vi "PictureMaquree.vi"() -> ()   [LabVIEW 2021]
uses:
  Control 1.ctl
  <vilib>/vision/NI_Vision_Development_Module.lvlib
panel:
  out "selected path":path
  in  "Delay Times":u64(knob) scale=1.0..500.0
  out "Original":T1(plugin-control)
  in  "Threshold":i64(slide)=125 scale=0.0..255.0
  out "Output Array":bool[][](array[boolean])
  out "ROI":T1(plugin-control)
  in  "Add Button":bool
  in  "Stop Button":bool
  in  "Pause Button":bool
  in  "Play Button":bool
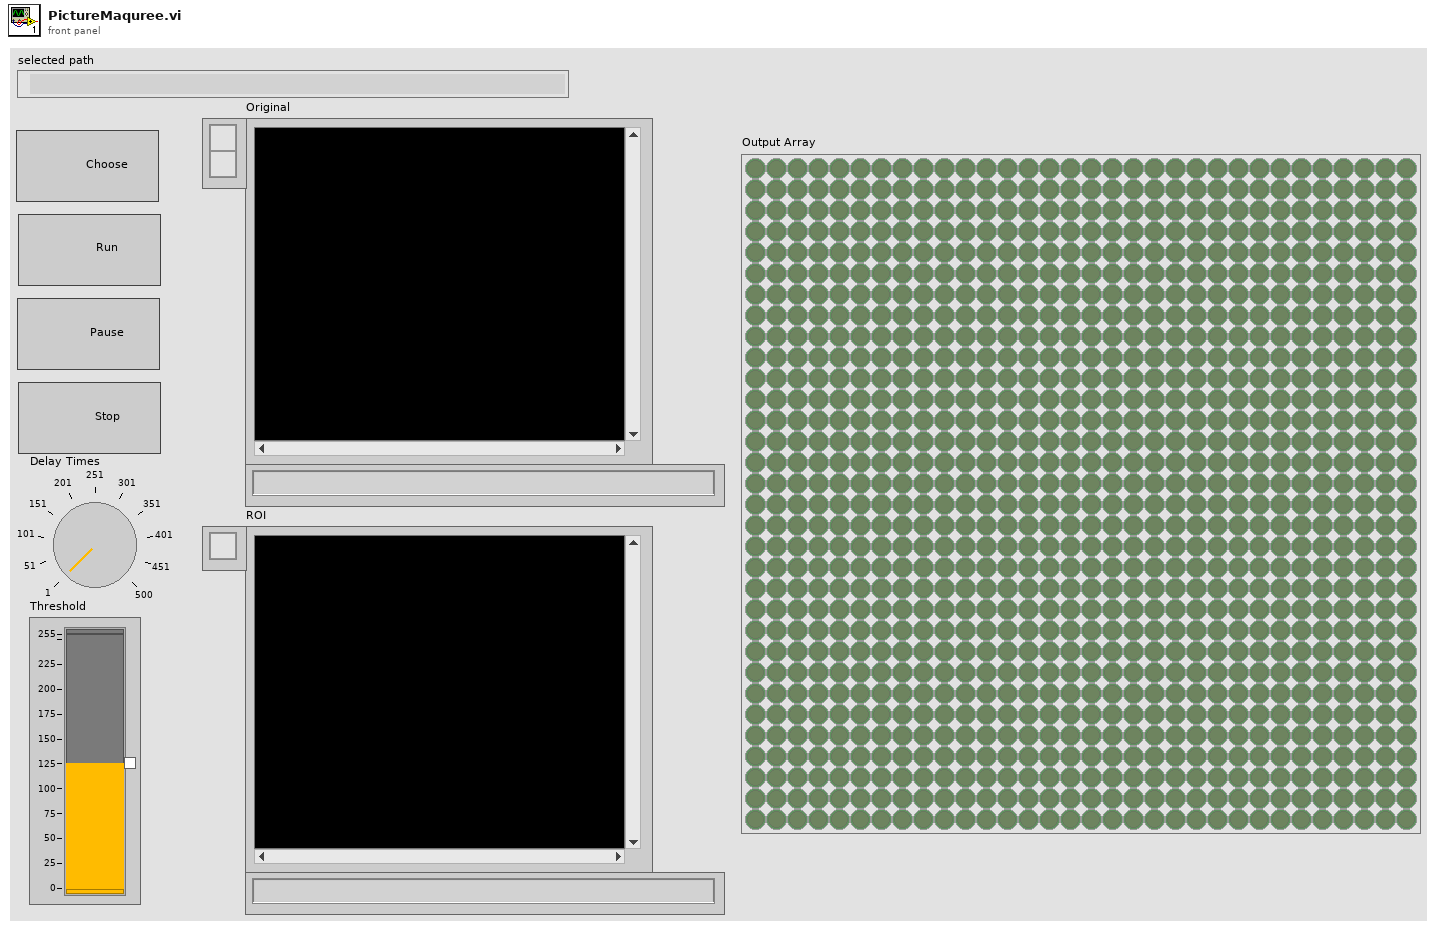
[diagram p1: front panel]
types:
  T1 = typedef "IMAQ Image.ctl" = refnum<image>
  T2 = typedef "Control 1.ctl" = enum16{"Initialize", "Open", "ROI", "Run", "Pause", "Stop"}
  T3 = typedef "Image Type" = u32
  T4 = cluster{"Global Rectangle":i32[], "Contours":cluster{"Contour Type":u32, "ROI Type":u32, "Points":i32[]}[]}
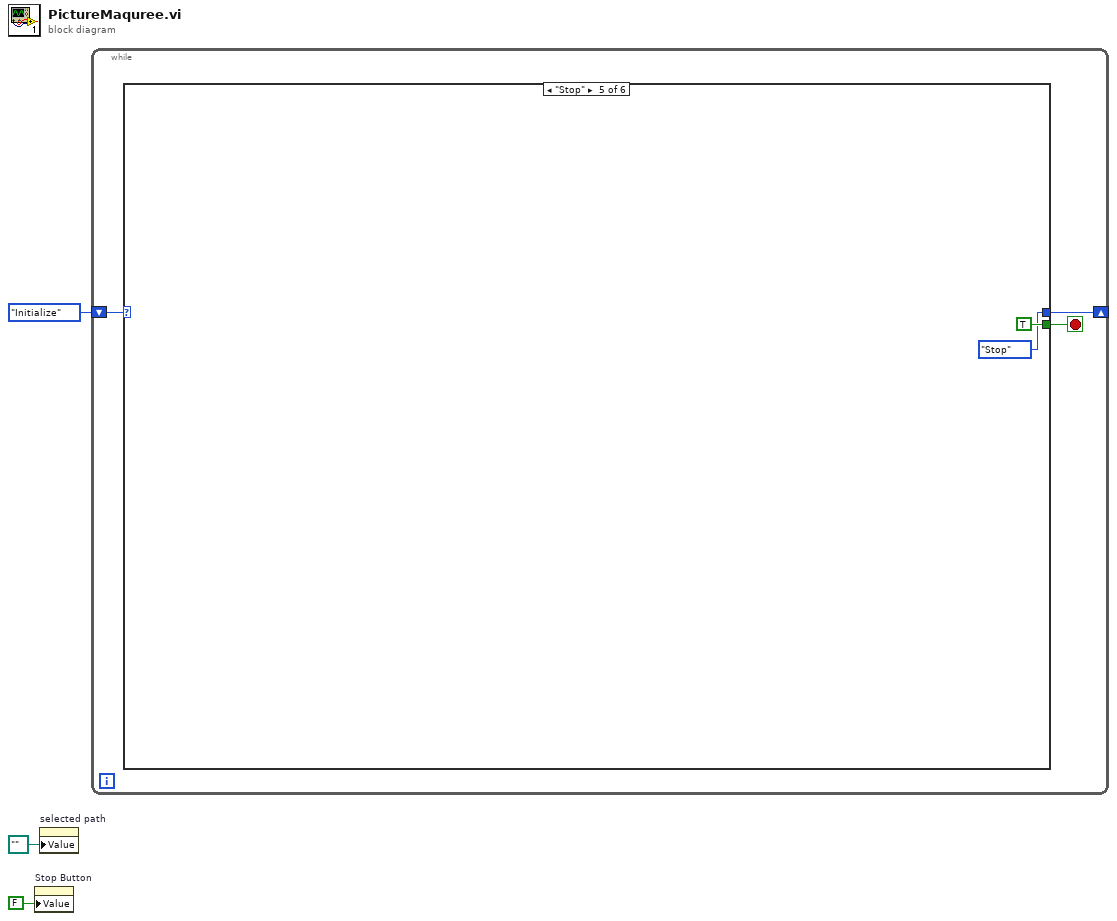
[diagram p0: block diagram]
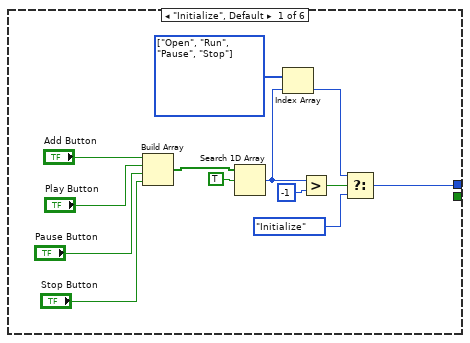
[diagram p2: hidden frame]
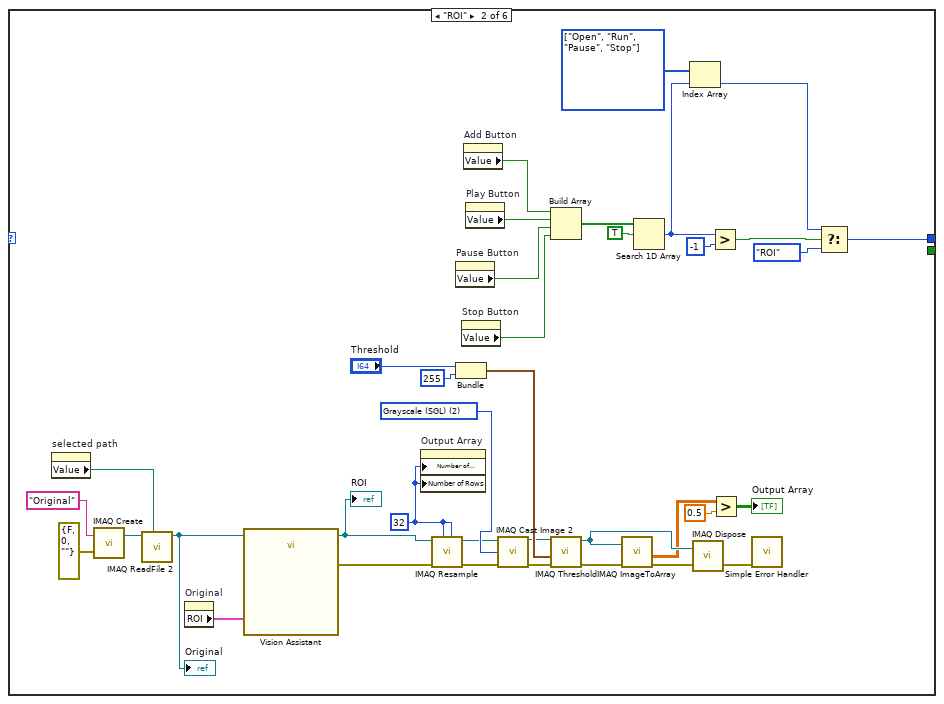
[diagram p3: hidden frame]
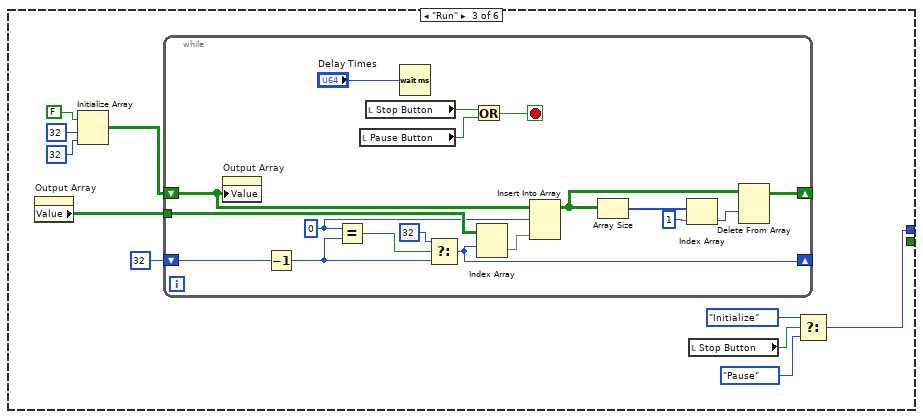
[diagram p4: hidden frame]
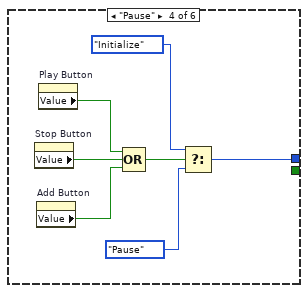
[diagram p5: hidden frame]
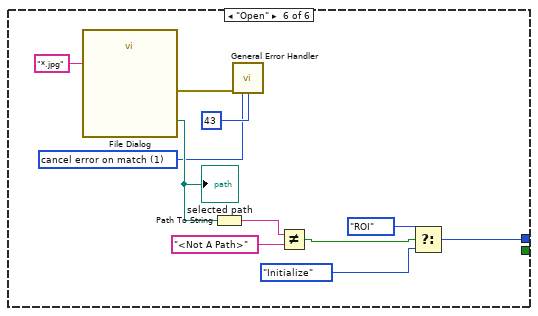
[diagram p6: hidden frame]
diagram:
  n1 = property on="Stop Button" class="Bool (strict)"("Value"=FALSE ("Stop Button")) -> ()  [unwired: 2 in, 2 out]
  n2 = property on="selected path" class="Path"("Value"=path "" ("selected path")) -> ()  [unwired: 2 in, 2 out]
  n3 = while {
    shift-right: [w5] -> _
    shift-left: Control_1."Initialize" -> [w4]
    stop <- w6 stop-if-true
    n4 = case shown="\"Stop\"" w4 {
      tunnel: [_ _ _ _ TRUE _] -> w6
      tunnel: [w10 w32 w64 w89 Control_1."Stop" w94] -> w5
      frame "Initialize", Default {
        w16 = T2[] [enum."Open", enum."Run", enum."Pause", enum."Stop"] items=["Initialize", "Open", "ROI", "Run", "Pause", "Stop"]
        n5 = Build Array("Add Button", "Play Button", "Pause Button", "Stop Button") -> (w18:bool[])
        n6 = Search 1D Array(1D array=w18, element=TRUE) -> (index of element=w12:i32)  [unwired: 1 in]
        n7 = Index Array(array=w16, index=w12) -> (element=w15:T2)
        n8 = Greater?(x=w12, y=-1) -> (0:w13:bool)
        n9 = Select(t=w15, s=w13, f=Control_1."Initialize") -> (s? t:f=w10:T2)
      }
      frame "ROI" {
        w25 = T2[] [enum."Open", enum."Run", enum."Pause", enum."Stop"] items=["Initialize", "Open", "ROI", "Run", "Pause", "Stop"]
        w33 = u32 32 ("Number of Rows")
        w50 = T3 2 items=["Grayscale (U8)", "Grayscale (I16)", "Grayscale (SGL)", "Complex (CSG)", "RGB (U32)", "HSL (U32)", "RGB (U64)", "Grayscale (U16)"] ("Image Type")
        n10 = property on="selected path" class="Path"() -> ("Value"=w53:path)  [unwired: 2 in, 2 out]
        n11 = call "IMAQ Create"("Image Name"="Original", "error in (no error)"=errorcluster {"status"=FALSE, "code"=0, "source"=""}) -> ("New Image"=w54:T1)  [unwired: 3 in, 1 out]
        n12 = call "IMAQ ReadFile 2"("File Path"=w53, "Image"=w54) -> ("Image Out"=w52:T1)  [unwired: 5 in, 4 out]
        "Original" <- w52
        n13 = property on="Original" class="ImageControl"() -> ("ROI"=w51:T4)  [unwired: 2 in, 2 out]
        n14 = call "Vision Assistant"("Image In"=w52, "ROI Descriptor (Image Mask 1)"=w51) -> ("Image Out"=w34:T1, "error out"=w47:errorcluster)  [unwired: 24 in]
        "ROI" <- w34
        n15 = property on="Output Array" class="Arr (strict)"("Number of Columns"=w33, "Number of Rows"=w33) -> ()  [unwired: 2 in, 2 out]
        n16 = call "IMAQ Resample"("X Resolution"=w33, "Y Resolution"=w33, "error in (no error)"=w47, "Image Src"=w34) -> ("error out"=w49:errorcluster, "Image Dst Out"=w48:T1)  [unwired: 6 in]
        n17 = property on="Pause Button" class="Bool (strict)"() -> ("Value"=w29:bool)  [unwired: 2 in, 2 out]
        n18 = Bundle("Threshold"="Threshold", 255) -> (w46:cluster{"Threshold":i64, i32})  [unwired: 1 in]
        n19 = property on="Stop Button" class="Bool (strict)"() -> ("Value"=w28:bool)  [unwired: 2 in, 2 out]
        n20 = property on="Add Button" class="Bool (strict)"() -> ("Value"=w31:bool)  [unwired: 2 in, 2 out]
        n21 = property on="Play Button" class="Bool (strict)"() -> ("Value"=w30:bool)  [unwired: 2 in, 2 out]
        n22 = call "IMAQ Cast Image 2"("Image Src"=w48, "Image Type"=w50, "error in (no error)"=w49) -> ("Image Dst Out"=w38:T1, "error out"=w37:errorcluster)  [unwired: 11 in]
        n23 = Build Array(w31, w30, w29, w28) -> (w27:bool[])
        n24 = call "IMAQ Threshold"("error in (no error)"=w37, "Range"=w46, "Image Src"=w38) -> ("error out"=w40:errorcluster, "Image Dst Out"=w42:T1)  [unwired: 7 in]
        n25 = call "IMAQ ImageToArray"("error in (no error)"=w40, "Image"=w42) -> ("Image Pixels (Float)"=w39:sgl[][], "error out"=w41:errorcluster)  [unwired: 2 in, 3 out]
        n26 = Search 1D Array(1D array=w27, element=TRUE) -> (index of element=w24:i32)  [unwired: 1 in]
        n27 = Index Array(array=w25, index=w24) -> (element=w21:T2)
        n28 = call "IMAQ Dispose"("Image"=w42, "error in (no error)"=w41) -> ("error out"=w43:errorcluster)  [unwired: 4 in]
        n29 = Greater?(x=w24, y=-1) -> (0:w22:bool)
        n30 = Greater?(x=w39, y=0.5) -> (0:→"Output Array":bool[][])
        n31 = call <vilib>:"Simple Error Handler.vi"("error in (no error)"=w43) -> ()  [unwired: 4 in, 5 out]
        n32 = Select(t=w21, s=w22, f=Control_1."ROI") -> (s? t:f=w32:T2)
      }
      frame "Run" {
        n33 = property on="Output Array" class="Arr (strict)"() -> ("Value"=w58:bool[][])  [unwired: 2 in, 2 out]
        n34 = Initialize Array(FALSE, 32 ("dimension size"), 32 ("dimension size")) -> (w59:bool[][])
        n35 = while {
          shift-right: [w67] -> _
          shift-left: w59 -> [w73]
          tunnel: w58 -> [w80]
          shift-right: [w75] -> _
          shift-left: 32 -> [w79]
          stop <- w82 stop-if-true
          w72 = 0 ("x")
          n36 = property on="Output Array" class="Arr (strict)"("Value"=w73) -> ()  [unwired: 2 in, 2 out]
          n37 = Decrement(x=w79) -> (x-1=w77:i32)
          n38 = Equal?(x=w72, y=w77) -> (x = y?=w76:bool)
          n39 = local read "Pause Button"() -> (w84:bool)
          n40 = local read "Stop Button"() -> (w83:bool)
          n41 = Wait (ms)(milliseconds to wait="Delay Times") -> ()  [unwired: 1 out]
          n42 = Select(t=32, s=w76, f=w77) -> (s? t:f=w75:i32)
          n43 = Or(x=w83, y=w84) -> (x .or. y?=w82:bool)
          n44 = Index Array(array=w80, index (row)=w75) -> (element=w74:bool[])  [unwired: 1 in]
          n45 = Insert Into Array(array=w73, index (row)=w72, new element=w74) -> (w69:bool[][])  [unwired: 1 in]
          n46 = Array Size(array=w69) -> (size(s)=w71:i32[])
          n47 = Index Array(array=w71, index=1) -> (element=w68:i32)
          n48 = Delete From Array(array=w69, index (row)=w68) -> (array with subset deleted=w67:bool[][])  [unwired: 2 in, 1 out]
        }
        n49 = local read "Stop Button"() -> (w63:bool)
        n50 = Select(t=Control_1."Initialize", s=w63, f=Control_1."Pause") -> (s? t:f=w64:T2)
      }
      frame "Pause" {
        n51 = property on="Stop Button" class="Bool (strict)"() -> ("Value"=w87:bool)  [unwired: 2 in, 2 out]
        n52 = property on="Add Button" class="Bool (strict)"() -> ("Value"=w85:bool)  [unwired: 2 in, 2 out]
        n53 = property on="Play Button" class="Bool (strict)"() -> ("Value"=w88:bool)  [unwired: 2 in, 2 out]
        n54 = Compound Arithmetic op=OR(w88, w87, w85) -> (w86:bool)
        n55 = Select(t=Control_1."Initialize", s=w86, f=Control_1."Pause") -> (s? t:f=w89:T2)
      }
      frame "Stop" {
      }
      frame "Open" {
        w98 = 1 items=["no exception", "cancel error on match", "set error on match"] ("[exception action] (none:0)")
        n56 = call "File Dialog"("pattern (all files)"="*.jpg") -> ("selected path"=w103:path, "error out"=w100:errorcluster)  [unwired: 11 in, 2 out]
        "selected path" <- w103
        n57 = Path To String(path=w103) -> (string=w102:string)
        n58 = call <vilib>:"General Error Handler.vi"("error in (no error)"=w100, "[exception action] (none:0)"=w98, "[exception code]"=43) -> ()  [unwired: 8 in, 5 out]
        n59 = Not Equal?(x=w102, y="<Not A Path>") -> (x != y?=w95:bool)
        n60 = Select(t=Control_1."ROI", s=w95, f=Control_1."Initialize") -> (s? t:f=w94:T2)
      }
    }
  }
